vi "Hexapod_GUI(old).vi"(10 "stop 2":refnum<vi>, 11 "GUI_cluster":T1={"Sub Panel"=refnum, "GUIdevice"="Bella_LP_Mode", "CtlRef"=refnum, "User Event in"=refnum}) -> ()   [LabVIEW 2013]
uses:
  Shared/GUI_Template/GUI_master/tcp_new_data_event.ctl
  Shared/GUI_Template/GUI_master/tcp new data cluster.ctl
  Controls/GUI_cluster.ctl
  Controls/eventtypdef1.ctl
panel:
  in  "<command>::1":bool
  in  "stepsize::1":dbl=0.02 caption="stepsize" min=0.0 max=10.0
  in  "relativemove.zpos::1":bool
  in  "relativemove.zneg::1":bool
  in  "wangle::1":dbl caption="w" min=-5.0 max=5.0
  in  "vangle::1":dbl caption="v" min=-5.0 max=5.0
  in  "uangle::1":dbl caption="u" min=-5.0 max=5.0
  in  "zpos::1":dbl=11.2 caption="z" min=-12.0 max=12.0
  in  "ypos::1":dbl=4.0 caption="y" min=-20.0 max=20.0
  in  "xpos::1":dbl=-1.0 caption="x" min=-20.0 max=20.0
  in  "relativemove.ypos::1":bool
  in  "relativemoveyneg::1":bool
  in  "relativemove.xneg::1":bool
  in  "relativemove.xpos::1":bool
  out "tcp data event":T2
  out "GUIdevice 1":string="StagingHexapodPI"
  in  "stop":bool
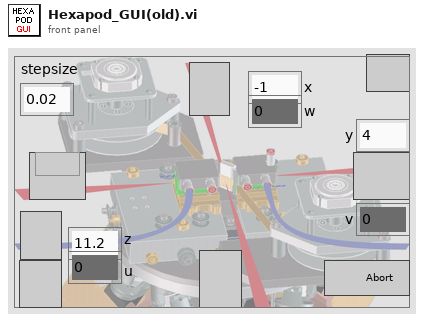
[diagram p1: front panel]
types:
  T1 = typedef "GUI_cluster.ctl" = cluster{"Sub Panel":refnum<vi>, "GUIdevice":string, "CtlRef":refnum<vi>, "User Event in":refnum<user-event>}
  T2 = typedef "tcp_new_data_event.ctl" = refnum<user-event>
  T3 = typedef "eventtypdef1.ctl" = cluster{"label":string, "Sub Panel":refnum<vi>, "CtlRef":refnum<vi>, "This VI":refnum<vi>}
  T4 = typedef "tcp new data cluster.ctl" = cluster{"EventEnum":enum16{"new data", "connection status update"}, "Device name":string}
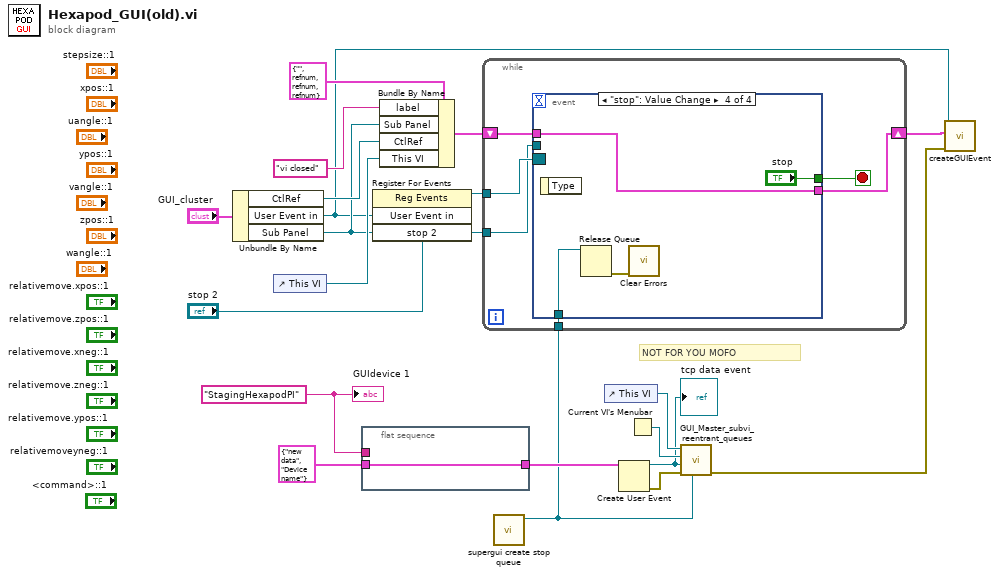
[diagram p0: block diagram]
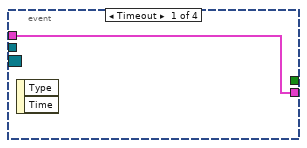
[diagram p2: hidden frame]
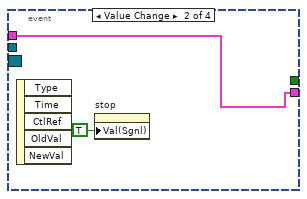
[diagram p3: hidden frame]
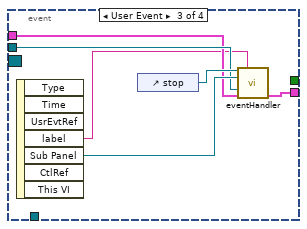
[diagram p4: hidden frame]
diagram:
  w10 = "StagingHexapodPI" ("GUIdevice")
  # "NOT FOR YOU MOFO"
  n1 = Unbundle By Name("GUI_cluster") -> ("CtlRef"=w12:refnum<vi>, "User Event in"=w5:refnum<user-event>, "Sub Panel"=w7:refnum<vi>)
  n2 = control-ref of="This VI"() -> (w11:refnum<vi>)
  n3 = flat-sequence {
    tunnel: T4 {"EventEnum"=enum."new data", "Device name"="Device name"} ("New Event") -> [w21]
    tunnel: [w21] -> w13
    tunnel: w10 -> [_]
    frame #0 {
    }
  }
  n4 = register-events(w5, "stop 2") -> (reference out=w9:refnum<event-registration>)  [unwired: 2 in, 1 out]
  n5 = Bundle By Name(cluster=T3 {"label"="", "Sub Panel"=refnum, "CtlRef"=refnum, "This VI"=refnum} ("event data"), "label"="vi closed", "Sub Panel"=w7, "CtlRef"=w12, "This VI"=w11) -> (w6:T3)
  n6 = call "supergui create stop queue.vi"() -> ("STOP Queue out"=w1:refnum<queue>)  [unwired: 11 in]
  n7 = while {
    tunnel: w9 -> [w27]
    tunnel: w7 -> [w25]
    shift-right: [w23] -> w3
    shift-left: w6 -> [w24]
    tunnel: w1 -> [w22]
    stop <- w26 stop-if-true
    n8 = event shown="[3] \"stop\": Value Change" {
      selector: w27 -> [_ _ _ _]
      dyn-events: _ -> [_ _ _ _]
      timeout: _ -> [_ _ _ _]
      tunnel: [_ _ _ "stop"] -> w26
      tunnel: w25 -> [_ _ w34 _]
      tunnel: w24 -> [w28 w30 w33 w39]
      tunnel: [w28 w30 w32 w39] -> w23
      tunnel: w22 -> [_ _ _ w38]
      event Timeout {
        n9 = event-data() -> ()  [unwired: 1 in, 2 out]
      }
      event Value Change {
        n10 = event-data() -> ()  [unwired: 1 in, 5 out]
        n11 = property on="stop" class="Bool (strict)"("Val(Sgnl)"=TRUE ("Value (Signaling)")) -> ()  [unwired: 2 in, 2 out]
      }
      event User Event {
        n12 = event-data() -> ("label"=w31:string, "Sub Panel"=w35:refnum<vi>)  [unwired: 1 in, 5 out]
        n13 = control-ref of="stop"() -> (w36:refnum<vi>)
        n14 = call "eventHandler.vi"("Boolean in"=w36, "label"=w31, "Sub Panel 2"=w35, "Sub Panel"=w34, "event data in"=w33) -> ("event data out"=w32:T3)  [unwired: 10 in]
      }
      event "stop": Value Change {
        n15 = event-data() -> ()  [unwired: 1 in, 1 out]
        n16 = Release Queue(queue=w38) -> (error out=w37:errorcluster)  [unwired: 2 in, 2 out]
        n17 = call <vilib>:"Clear Errors.vi"("error in (no error)"=w37) -> ()  [unwired: 6 in, 1 out]
      }
    }
  }
  n18 = control-ref of="This VI"() -> (w20:refnum<vi>)
  n19 = Create User Event(user event datatype=w13) -> (user event=w17:refnum<user-event>, error out=w18:errorcluster)  [unwired: 1 in]
  "tcp data event" <- w17
  n20 = Current VI's Menubar() -> (w19:refnum<k9>)
  n21 = call "GUI_Master_subvi_reentrant_queues.vi"("STOP Queue in"=w1, "error in (no error)"=w18, "tcp data event"=w17, "Caller menu reference"=w19, "Caller VI ref"=w20) -> ("error out"=w4:errorcluster)  [unwired: 6 in]
  n22 = call "createGUIEvent.vi"("error in (no error)"=w4, "event data"=w3, "User Event in"=w5) -> ()  [unwired: 8 in, 1 out]
  "GUIdevice 1" <- w10
